vi "delete Test.vi"(8 "error in (no error)":errorcluster caption="Fehler (Eingang, kein Fehler)", 10 "index":i32 caption="Index", 11 "Report (Eingang)":refnum<class "Report.lvclass">) -> (0 "error out":errorcluster caption="Fehler (Ausgang)", 3 "Report (Ausgang)":refnum<class "Report.lvclass">)   [LabVIEW 2013, in "DatenKlassen.lvlib" / "Report.lvclass"]
uses:
  Report.lvclass
  Report.lvclass/Report.ctl
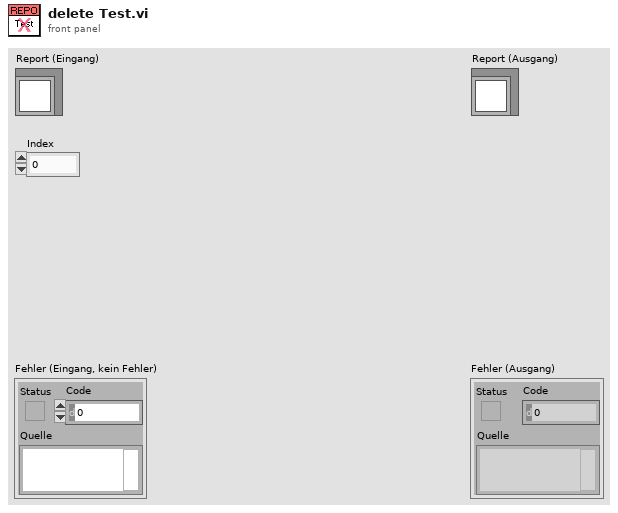
[diagram p1: front panel]
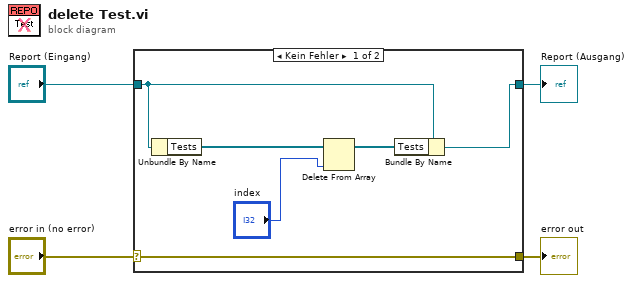
[diagram p0: block diagram]
diagram:
  n1 = case shown="Kein Fehler" "error in (no error)" {
    selector: "error in (no error)" -> [w10 w11]
    tunnel: [w10 w11] -> w3
    tunnel: [w9 w12] -> w1
    tunnel: "Report (Eingang)" -> [w8 w12]
    frame No Error {
      n2 = Unbundle By Name(w8) -> ("Tests"=w7:refnum<class "Test.lvclass">[])
      n3 = Delete From Array(array=w7, index="index") -> (array with subset deleted=w6:refnum<class "Test.lvclass">[])  [unwired: 1 in, 1 out]
      n4 = Bundle By Name(cluster=w8, "Tests"=w6) -> (w9:refnum<class "Report.lvclass">)
    }
    frame Error {
    }
  }
  "error out" <- w3
  "Report (Ausgang)" <- w1
